vi "App Builder.vi"(2 "error in (no error)":errorcluster, 3 "Path":path) -> (0 "error out":errorcluster, 1 "Generated files":path[](array[path]))   [LabVIEW 2014]
uses:
  <vilib>/AppBuilder/AB_API_Simple/Build (path).vi
  <vilib>/AppBuilder/AB_API_Simple/NI_App_Builder_API.lvlib
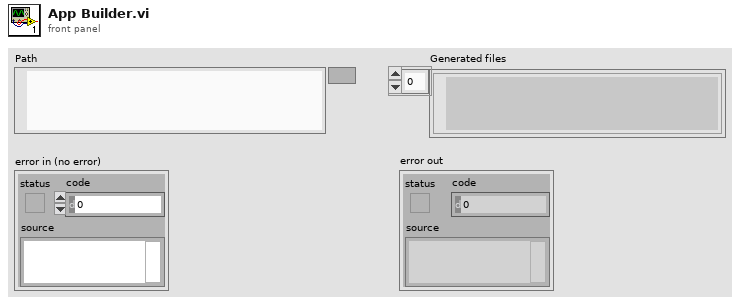
[diagram p1: front panel]
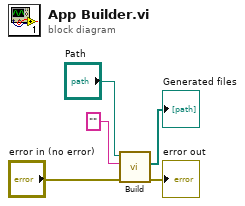
[diagram p0: block diagram]
diagram:
  n1 = call-poly <vilib>:"Build.vi"("error in (no error)"="error in (no error)", "Name of build specification (if empty: build all)"="", "Path to project"="Path") -> ("error out"=→"error out":errorcluster, "Generated files"=→"Generated files":path[])  [unwired: 7 in]
